vi "Save Settings.vi"(8 "error in (no error)":errorcluster {"code" format="Error %.0f"}, 11 "VIDoc Settings - Confluence In":refnum<class "VIDoc Settings - Confluence.lvclass">) -> (0 "error out":errorcluster {"code" format="Error %.0f"}, 3 "VIDoc Settings - Confluence Out":refnum<class "VIDoc Settings - Confluence.lvclass">)   [LabVIEW 2023, in "VIDoc Printer - Confluence.lvlib" / "VIDoc Settings - Confluence.lvclass"]
uses:
  VIDoc Settings - Confluence.lvclass
  C:/projects/DMC/Tooling/Git-Action-Service/Source/Documentation Generation/Settings/VIDoc Settings/VIDoc Settings.lvclass
  VIDoc Settings - Confluence.lvclass/VIDoc Settings - Confluence.ctl
  VIDoc Settings/VIDoc Settings.lvclass/VIDoc Settings.ctl
  VIDoc Settings/Get VIDoc Settings Path.vi
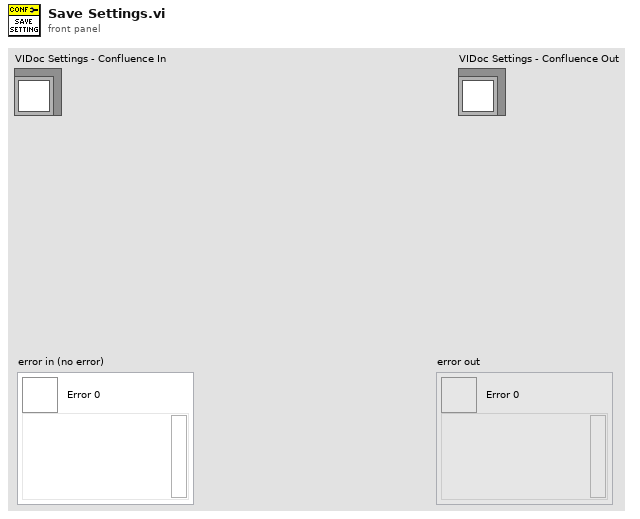
[diagram p1: front panel]
types:
  T1 = typedef "VIDoc Printer - Confluence.lvlib/VIDoc Settings - Confluence.lvclass/Confluence Connection Settings.ctl" = cluster{"Connection Type":enum16{"Data Center", "Cloud"}, "URL":string, "Email":string}
  T2 = typedef "VIDoc Printer - Confluence.lvlib/VIDoc Settings - Confluence.lvclass/Confluence Printer Settings Cluster.ctl" = cluster{"Expand Structures":cluster{"VI Member":cluster{"By Folder Expand":bool, "By Tree Expand":bool, "By List Expand":bool, "Methods Expand":bool, "Controls Expand":bool}, "Control Member":cluster{"By Folder Expand":bool, "By Tree Expand":bool, "By List Expand":bool, "Controls Expand":bool}, "Interface":cluster{"List Expand":bool, "Controls Expand":bool, "Methods Expand":bool, "Inheritance Expand":bool}, "Library":cluster{"By Folder Expand":bool, "By Tree Expand":bool, "By List Expand":bool, "Controls Expand":bool, "Methods Expand":bool, "Inheritance Expand":bool}, "Class":cluster{"By Folder Expand":bool, "By Tree Expand":bool, "By List Expand":bool, "CPD Expand":bool, "Controls Expand":bool, "Methods Expand":bool, "Set Accessors Expand":bool, "Get Accessors Expand":bool, "Inheritance Expand":bool}}, "Sortable Tables":bool, "Table Column Ordering":cluster{"Class List":cluster{"Minimal":T3[], "Standard":T3[], "Full":T3[]}, "Library List":cluster{"Minimal":T3[], "Standard":T3[], "Full":T3[]}, "Control FP":cluster{"Minimal":T4[], "Standard":T4[], "Full":T4[]}, "Library Control Files":cluster{"Minimal":T5[], "Standard":T5[], "Full":T5[]}, "UI Methods":cluster{"Minimal":T5[], "Standard":T5[], "Full":T5[]}, "Method List":cluster{"Minimal":T5[], "Standard":T5[], "Full":T5[]}, "Interface Methods":cluster{"Minimal":T5[], "Standard":T5[], "Full":T5[]}, "LLB Methods":cluster{"Minimal":T5[], "Standard":T5[], "Full":T5[]}, "Library Methods":cluster{"Minimal":T5[], "Standard":T5[], "Full":T5[]}, "Class Methods":cluster{"Minimal":T5[], "Standard":T5[], "Full":T5[]}}}
  T3 = typedef "VIDoc Printer - Confluence.lvlib/VIDoc Settings - Confluence.lvclass/Class Info Column.ctl" = enum16{"Image", "Name", "Description", "Version", "Last Change", "Author", "Commit Hash", "Branch", "Qualified Name", "TransferMustOverrides", "ChildRefsRestricted"}
  T4 = typedef "VIDoc Printer - Confluence.lvlib/VIDoc Settings - Confluence.lvclass/Control Info Column.ctl" = enum16{"Image", "Name", "Description", "Caption", "Tip Strip", "Data Type", "Key Toggle"}
  T5 = typedef "VIDoc Printer - Confluence.lvlib/VIDoc Settings - Confluence.lvclass/VI Info Column.ctl" = enum16{"Name", "Conpane", "BD", "FP", "VI Icon", "Description", "Reentrant", "Inline", "Auto Error", "Compiled", "Code Complexity", "Data Size", "Debug", "Priority", "Rev", "Minimum Size", "Title", "FP Behavior", "FP Closeable", "Author", "Commit Hash", "Last Change", "Branch", "Scope", "Type", "Dispatch", "Must Override", "Must Use Parent", "Structure Tree"}
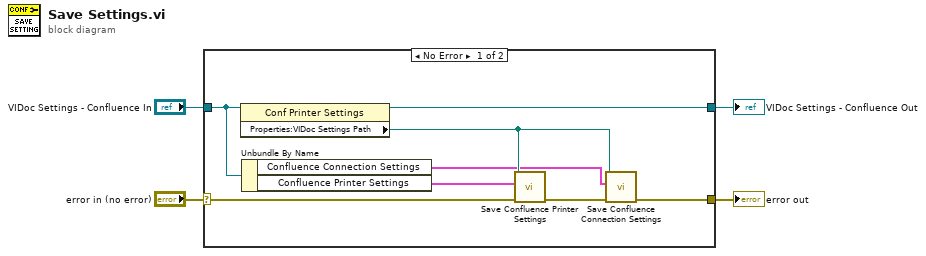
[diagram p0: block diagram]
diagram:
  n1 = case shown="No Error" "error in (no error)" {
    selector: "error in (no error)" -> [w11 w14]
    tunnel: [w10 w14] -> w3
    tunnel: [w9 w13] -> w2
    tunnel: "VIDoc Settings - Confluence In" -> [w7 w13]
    frame No Error {
      n2 = property class="Conf Printer Settings"(reference=w7) -> (reference out=w9:refnum<class "VIDoc Settings - Confluence.lvclass">, "Properties:VIDoc Settings Path"=w8:path)  [unwired: 1 in, 1 out]
      n3 = Unbundle By Name(w7) -> ("Confluence Connection Settings"=w6:T1, "Confluence Printer Settings"=w5:T2)
      n4 = call "Save Confluence Printer Settings.vi"("Error in"=w11, "Confluence Printer Settings"=w5, "Settings Path"=w8) -> ("Error out"=w12:errorcluster)  [unwired: 8 in]
      n5 = call "Save Confluence Connection Settings.vi"("Error in"=w12, "Confluence Connection Settings"=w6, "Settings Path"=w8) -> ("Error out"=w10:errorcluster)  [unwired: 8 in]
    }
    frame Error {
    }
  }
  "error out" <- w3
  "VIDoc Settings - Confluence Out" <- w2
